vi "Smooth_Data.vi"(0 "Plot cluster":cluster{"Xo":dbl, "Delta X":dbl, dbl[]} {"?" format="%.2f"; "Delta X" format="%.2f"; "Xo" format="%.2f"}, 7 "Plot type":string, 9 "OK":bool, 11 "Trace name":string, 12 "Trace No":i32) -> (4 "X array Out":dbl[](array[numeric]) format="%.2f", 8 "Y array Out":dbl[](array[numeric]) format="%.2f")   [LabVIEW 2010]
uses:
  Globals/Meas_global.vi
panel:
  in  "Save in separate files?":bool=TRUE
  in  "Use Whole Input Array":bool=TRUE
  in  "Y axis":cluster{"Mapping":u16, "Format":u16} {"Format" items=["Decimal", "Scientific", "Engineering"]; "Mapping" items=["Linear", "Logarithmic"]}
  in  "X axis":cluster{"Mapping":u16, "Format":u16} {"Format" items=["Decimal", "Scientific", "Engineering"]; "Mapping" items=["Linear", "Logarithmic"]}
  out "Raw data array size":i32
  out "Smoothed array size":i32
  in  "End index":i32
  in  "Start Index":i32
  in  "Smoothing":enum16{"Linear", "Logarithmic"}(ring)
  out "X,Y plot":cluster{dbl[], dbl[]}[](graph)
  in  "Number of smoothed estimates":i32=1
  # "Raw data array controls"
  # "Smoothing controls"
  # "Desired number of estimates"
  # "Spacing"
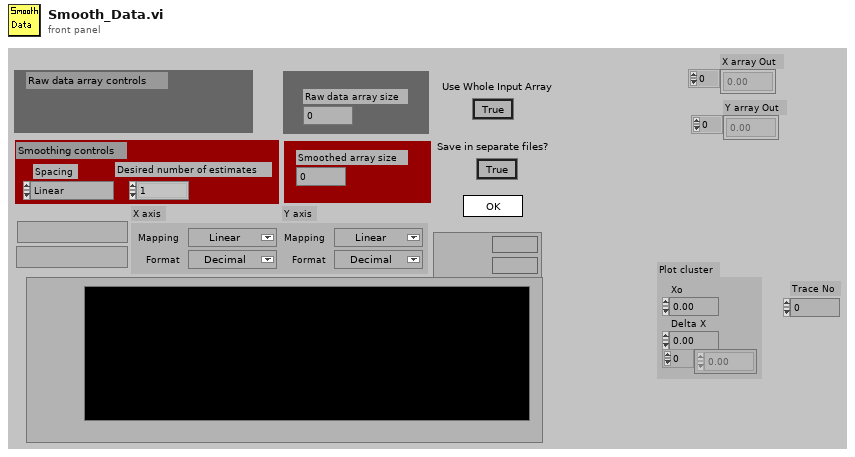
[diagram p1: front panel]
types:
  T1 = cluster{"Start Index":i32, "End Index":i32, "Smoothing":enum16{"Linear", "Logarithmic"}, "Number of smoothed estimates":i32, "X axis":cluster{"Mapping":u16, "Format":u16}, "Y axis":cluster{"Mapping":u16, "Format":u16}, "Use Whole Input Array?":bool}[]
  T2 = cluster{"Start Index":i32, "End Index":i32, "Smoothing":enum16{"Linear", "Logarithmic"}, "Number of smoothed estimates":i32, "X axis":cluster{"Mapping":u16, "Format":u16}, "Y axis":cluster{"Mapping":u16, "Format":u16}, "Use Whole Input Array?":bool}
  T3 = cluster{"X array Out":dbl[], "Y array Out":dbl[]}
  T4 = cluster{"X array Out":dbl[], "Y array Out":dbl[]}[]
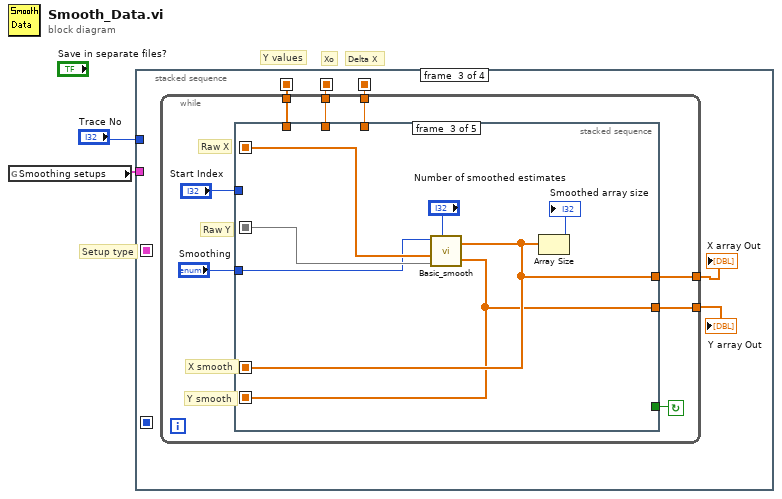
[diagram p0: block diagram]
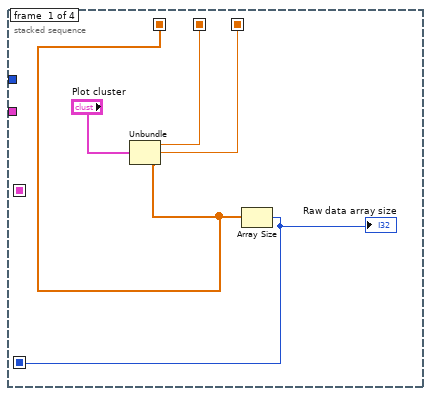
[diagram p2: hidden frame]
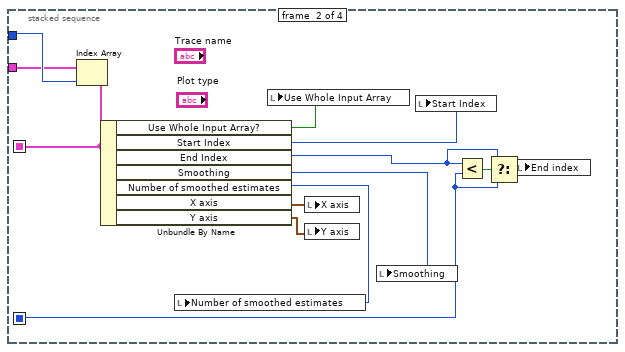
[diagram p3: hidden frame]
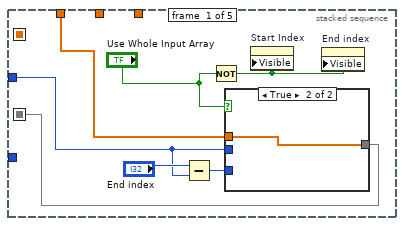
[diagram p4: hidden frame]
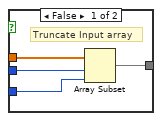
[diagram p5: hidden frame]
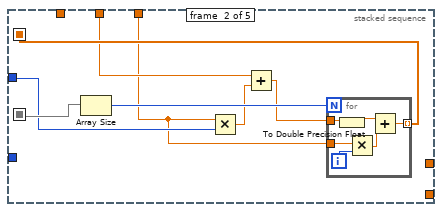
[diagram p6: hidden frame]
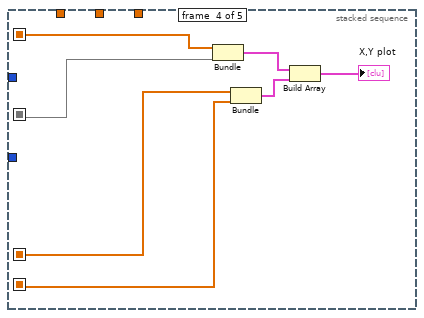
[diagram p7: hidden frame]
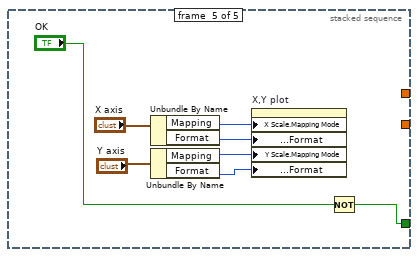
[diagram p8: hidden frame]
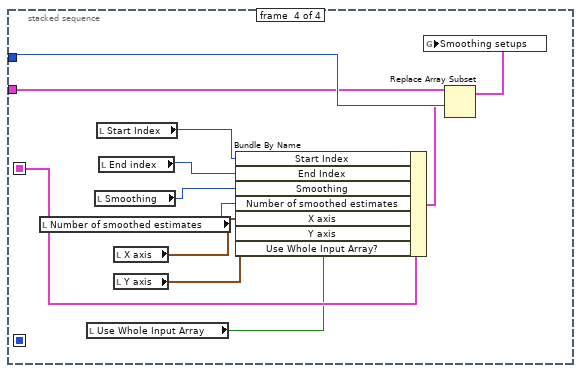
[diagram p9: hidden frame]
diagram:
  # "Setup type"
  # "Y values"
  # "Delta X"
  # "Xo"
  n1 = global read "Meas_global.vi" "Smoothing setups"() -> (w1:T1)
  n2 = stacked-sequence {
    seq-local: [w6 _ _ _] -> [_ _ w25 _]
    seq-local: [w5 _ _ _] -> [_ _ w24 _]
    seq-local: [w4 _ _ _] -> [_ w18 _ _]
    seq-local: [w3 _ _ _] -> [_ _ w23 _]
    seq-local: [_ w12 _ _] -> [_ _ _ w93]
    tunnel: "Trace No" -> [_ w16 _ w88]
    tunnel: w1 -> [_ w11 _ w86]
    frame #0 {
      n3 = Unbundle("Plot cluster") -> ("Xo"=w6:dbl, "Delta X"=w5:dbl, w3:dbl[])
      n4 = Array Size(array=w3) -> (size(s)=w4:i32)
      "Raw data array size" <- w4
    }
    frame #1 {
      n5 = Index Array(array=w11, index=w16) -> (element=w12:T2)
      n6 = Unbundle By Name(w12) -> ("Use Whole Input Array?"=w8:bool, "Start Index"=w15:i32, "End Index"=w14:i32, "Smoothing"=w13:enum16{"Linear", "Logarithmic"}, "Number of smoothed estimates"=w20:i32, "X axis"=w10:cluster{"Mapping":u16, "Format":u16}, "Y axis"=w9:cluster{"Mapping":u16, "Format":u16})
      n7 = local write "Number of smoothed estimates"(w20) -> ()
      n8 = local write "Use Whole Input Array"(w8) -> ()
      n9 = local write "X axis"(w10) -> ()
      n10 = local write "Y axis"(w9) -> ()
      n11 = local write "Smoothing"(w13) -> ()
      n12 = local write "Start Index"(w15) -> ()
      n13 = Less?(x=w14, y=w18) -> (x < y?=w19:bool)
      n14 = Select(t=w14, s=w19, f=w18) -> (s? t:f=w17:i32)
      n15 = local write "End index"(w17) -> ()
    }
    frame #2 {
      n16 = while {
        tunnel: w23 -> [w26]
        tunnel: w24 -> [w27]
        tunnel: w25 -> [w28]
        tunnel: [w30] -> w22
        tunnel: [w31] -> w21
        stop <- w32 continue-if-true
        # "Raw Y"
        # "Raw X"
        # "X smooth"
        # "Y smooth"
        n17 = stacked-sequence {
          seq-local: [w40 _ _ _ _] -> [_ w52 w64 w71 _]
          seq-local: [_ _ w61 _ _] -> [_ _ _ w68 _]
          seq-local: [_ _ w62 _ _] -> [_ _ _ w69 _]
          seq-local: [_ w53 _ _ _] -> [_ _ w65 w72 _]
          tunnel: "Start Index" -> [w37 w50 _ _ _]
          tunnel: [_ _ _ _ w81] -> w32
          tunnel: [_ _ w62 _ _] -> w31
          tunnel: [_ _ w61 _ _] -> w30
          tunnel: "Smoothing" -> [_ _ w60 _ _]
          tunnel: w28 -> [_ w47 _ _ _]
          tunnel: w27 -> [_ w46 _ _ _]
          tunnel: w26 -> [w39 _ _ _ _]
          frame #0 {
            n18 = Subtract(x="End index", y=w37) -> (x-y=w36:i32)
            n19 = Not(x="Use Whole Input Array") -> (.not. x?=w34:bool)
            n20 = case shown="True" "Use Whole Input Array" {
              tunnel: [w44 w45] -> w40
              tunnel: w39 -> [w43 w45]
              tunnel: w37 -> [w42 _]
              tunnel: w36 -> [w41 _]
              frame False {
                # "Truncate Input array"
                n21 = Array Subset(array=w43, index=w42, length=w41) -> (w44:dbl[])
              }
              frame True {
              }
            }
            n22 = property on="Start Index" class="DigNum (strict)"("Visible"=w34) -> ()  [unwired: 2 in, 2 out]
            n23 = property on="End index" class="DigNum (strict)"("Visible"=w34) -> ()  [unwired: 2 in, 2 out]
          }
          frame #1 {
            n24 = Array Size(array=w52) -> (size(s)=w51:i32)
            n25 = Multiply(x=w46, y=w50) -> (x*y=w49:dbl)
            n26 = Add(x=w47, y=w49) -> (x+y=w48:dbl)
            n27 = for {
              N: w51 -> [_]
              tunnel: w48 -> [w58]
              tunnel: w46 -> [w57]
              tunnel: [w54] -> w53 mode=indexing
              i -> [w56]
              n28 = To Double Precision Float(number=w58) -> (double precision float=w59:dbl)
              n29 = Multiply(x=w57, y=w56) -> (x*y=w55:dbl)
              n30 = Add(x=w59, y=w55) -> (x+y=w54:dbl)
            }
          }
          frame #2 {
            n31 = call "Basic_smooth.vi"("Smoothing"=w60, "X array in"=w65, "Y array in"=w64, "No of estimates output"="Number of smoothed estimates") -> ("X array Out"=w62:dbl[], "Y array Out"=w61:dbl[])  [unwired: 1 out]
            n32 = Array Size(array=w62) -> (size(s)=→"Smoothed array size":i32)
          }
          frame #3 {
            n33 = Bundle(w72, w71) -> (w70:cluster{dbl[], dbl[]})  [unwired: 1 out]
            n34 = Bundle("X array Out"=w69, "Y array Out"=w68) -> (w67:T3)  [unwired: 1 out]
            n35 = Build Array(w70, w67) -> (→"X,Y plot":T4)
          }
          frame #4 {
            n36 = Unbundle By Name("X axis") -> ("Mapping"=w78:u16, "Format"=w77:u16)
            n37 = Unbundle By Name("Y axis") -> ("Mapping"=w75:u16, "Format"=w74:u16)
            n38 = property on="X,Y plot" class="XYGraph (strict)"("X Scale.Mapping Mode"=w78, "X Scale.Format & Precision:Format"=w77, "Y Scale.Mapping Mode"=w75, "Y Scale.Format & Precision:Format"=w74) -> ()  [unwired: 2 in, 2 out]
            n39 = Not(x="OK") -> (.not. x?=w81:bool)
          }
        }
      }
      "X array Out" <- w21
      "Y array Out" <- w22
    }
    frame #3 {
      n40 = local read "Number of smoothed estimates"() -> (w89:i32)
      n41 = local read "Use Whole Input Array"() -> (w82:bool)
      n42 = local read "Smoothing"() -> (w90:enum16{"Linear", "Logarithmic"})
      n43 = local read "Start Index"() -> (w92:i32)
      n44 = local read "End index"() -> (w91:i32)
      n45 = local read "X axis"() -> (w84:cluster{"Mapping":u16, "Format":u16})
      n46 = local read "Y axis"() -> (w83:cluster{"Mapping":u16, "Format":u16})
      n47 = Bundle By Name(cluster=w93, "Start Index"=w92, "End Index"=w91, "Smoothing"=w90, "Number of smoothed estimates"=w89, "X axis"=w84, "Y axis"=w83, "Use Whole Input Array?"=w82) -> (w87:T2)
      n48 = Replace Array Subset(array=w86, new element=w87, index=w88) -> (w85:T1)
      n49 = global write "Meas_global.vi" "Smoothing setups"(w85) -> ()
    }
  }
